vi "Actor Core.vi"(8 "error in":errorcluster, 11 "HIJ Multiple Cams App Demo In":refnum<class "HIJ Multiple Cams App Demo.lvclass">) -> (0 "error out":errorcluster, 3 "Actor out":refnum<class "Actor.lvclass">)   [LabVIEW 2014, in "HIJ Multiple Cams App Demo.lvlib" / "HIJ Multiple Cams App Demo.lvclass"]
doc: "(<B>Filename</B>: Actor Framework.lvlib:Actor.lvclass:Actor Core.vi)\n\nReceives messages to the actor, reacts to them, and initiates any error handling that may shut the actor down.\n\nDescendant classes may override this VI to append parallel tasks for the actor to complete while it handles messages. Overrides use the Call Parent Method node."
uses:
  HIJ Multiple Cams App Demo.lvclass
  <vilib>/ActorFramework/Actor/Actor.lvclass
  Applications/HIJ Single Cam App Demo/HIJ Single Cam App Demo/HIJ Single Cam App Demo.lvclass
  HIJ Multiple Cams App Demo Messages/Results from Cam 1 Msg/Results from Cam 1 Msg.lvclass
  HIJ Multiple Cams App Demo Messages/Results from Cam 2 Msg/Results from Cam 2 Msg.lvclass
  Shared Code/Viewable Actor/ViewableActor/ViewableActor.lvclass/ViewableActor.ctl
  HIJ Multiple Cams App Demo.lvclass/HIJ Multiple Cams App Demo.ctl
  Applications/HIJ Single Cam App Demo/HIJ Single Cam App Demo/HIJ Single Cam App Demo.lvclass/HIJ Single Cam App Demo.ctl
  Shared Code/Viewable Actor/ViewableActor Messages/Insert Into SubPanel Msg/Insert Into SubPanel Msg.lvclass/Insert Into SubPanel Msg.ctl
  <vilib>/ActorFramework/Message Enqueuer/Message Enqueuer.lvclass/Message Enqueuer.ctl
  <vilib>/ActorFramework/Actor/Actor.lvclass/Actor.ctl
  Applications/HIJ Vision Camera App/HIJ Vision Camera App Messages/Menu Selection Msg/Menu Selection Msg.lvclass/Menu Selection Msg.ctl
  Shared Code/Viewable Actor/ViewableActor/Write UI VI Ref.vi
  Applications/HIJ Single Cam App Demo/HIJ Single Cam App Demo/Write Caller Menu Ref.vi
  Applications/HIJ Single Cam App Demo/HIJ Single Cam App Demo/Write Publish Analyze Results Msg.vi
  <vilib>/ActorFramework/Message Enqueuer/Enqueue.vi
  <vilib>/ActorFramework/Message Enqueuer/Init from Existing Queue.vi
  Applications/HIJ Vision Camera App/HIJ Vision Camera App/Write my WorkDir.vi
  Applications/HIJ Vision Camera App/HIJ Vision Camera App/Write my ConfigDir.vi
  Applications/HIJ Vision Camera App/HIJ Vision Camera App/Write Start Camera.vi
  Applications/HIJ Vision Camera App/HIJ Vision Camera App/Write Start Acquisition.vi
  <vilib>/ActorFramework/Message Priority Queue/Priority Enqueue.vi
  Shared Code/Viewable Actor/ViewableActor Messages/Insert Into SubPanel Msg/Insert Into SubPanel Msg.lvclass
  <vilib>/ActorFramework/Message Enqueuer/Message Enqueuer.lvclass
  Applications/HIJ Vision Camera App/HIJ Vision Camera App Messages/Menu Selection Msg/Menu Selection Msg.lvclass
  <vilib>/ActorFramework/Stop Msg/Stop Msg.lvclass
  Shared Code/Viewable Actor/ViewableActor/ViewableActor.lvclass
panel:
  in  "Stop Button":bool
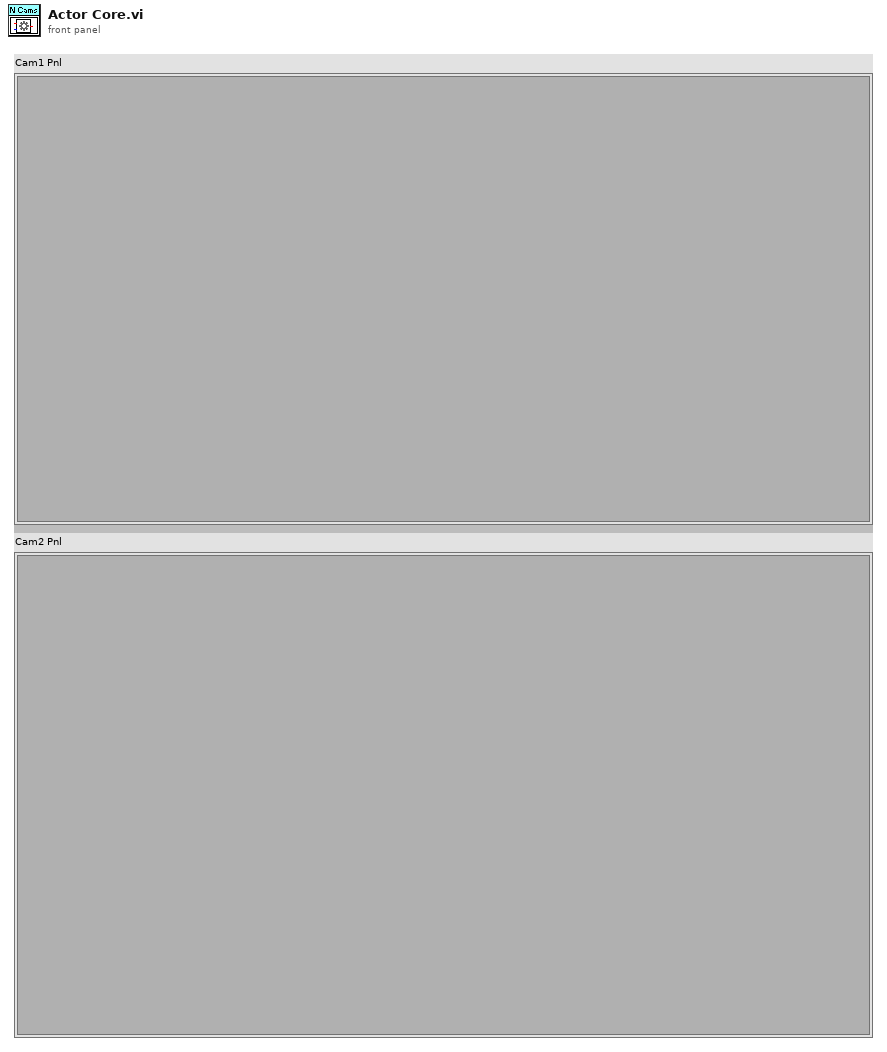
[diagram p1: front panel]
types:
  T1 = typedef "IMAQdx.ctl" = refnum<k21>
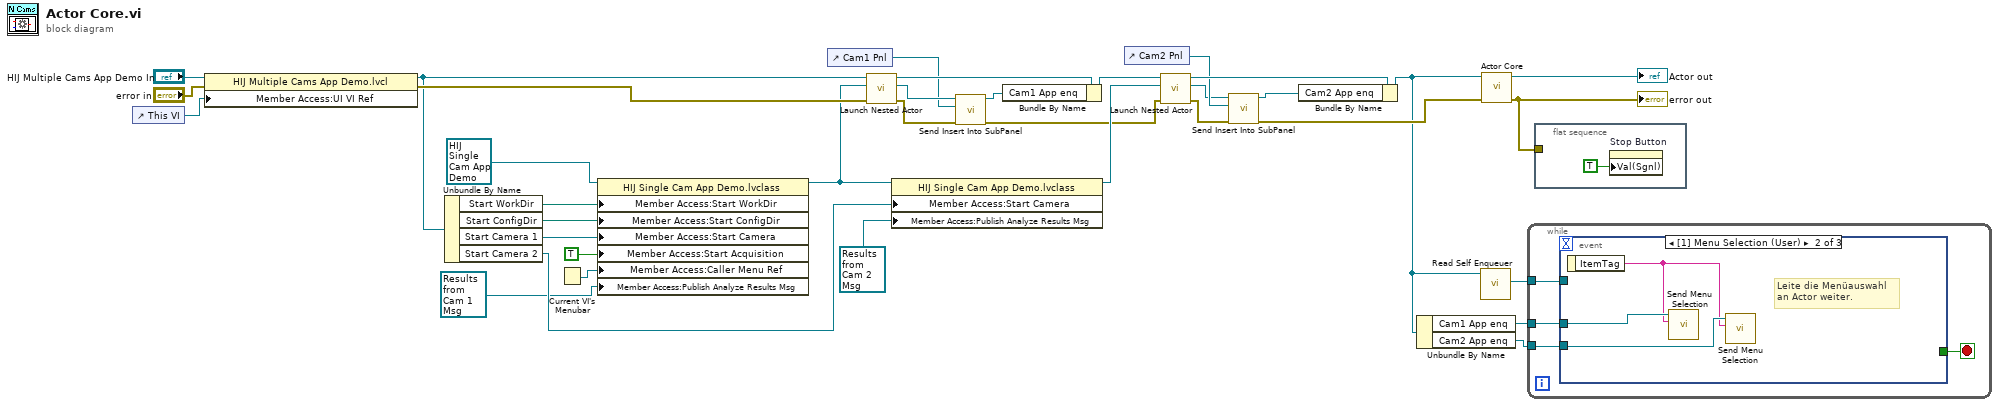
[diagram p0: block diagram]
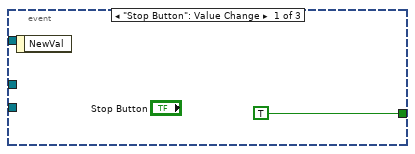
[diagram p2: hidden frame]
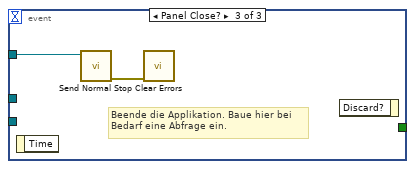
[diagram p3: hidden frame]
diagram:
  n1 = control-ref of="This VI"() -> (w30:refnum<vi>)
  n2 = property class="HIJ Multiple Cams App Demo.lvcl"(reference="HIJ Multiple Cams App Demo In", error in="error in", "Member Access:UI VI Ref"=w30) -> (reference out=w18:refnum<class "HIJ Multiple Cams App Demo.lvclass">, error out=w27:errorcluster)
  n3 = Unbundle By Name(w18) -> ("Start WorkDir"=w15:path, "Start ConfigDir"=w16:path, "Start Camera 1"=w17:T1, "Start Camera 2"=w14:T1)
  n4 = Current VI's Menubar() -> (w11:refnum<k9>)
  n5 = property class="HIJ Single Cam App Demo.lvclass"(reference=refnum<class "HIJ Single Cam App Demo.lvclass"> refnum ("HIJ Single Cam App Demo.lvlib:HIJ Single Cam App Demo.lvclass"), "Member Access:Start WorkDir"=w15, "Member Access:Start ConfigDir"=w16, "Member Access:Start Camera"=w17, "Member Access:Start Acquisition"=TRUE ("Start Acquisition"), "Member Access:Caller Menu Ref"=w11, "Member Access:Publish Analyze Results Msg"=refnum<class "Results from Cam 1 Msg.lvclass"> refnum ("HIJ Multiple Cams App Demo.lvlib:Results from Cam 1 Msg.lvclass")) -> (reference out=w26:refnum<class "HIJ Single Cam App Demo.lvclass">)  [unwired: 1 in, 1 out]
  n6 = control-ref of="Cam1 Pnl"() -> (w19:refnum<vi>)
  n7 = call <vilib>:"Launch Nested Actor.vi"("error in (no error)"=w27, "Nested Actor"=w26, "Caller Actor in"=w18) -> ("error out"=w22:errorcluster, "Nested Actor's Enqueuer"=w24:refnum<class "Message Enqueuer.lvclass">, "Caller Actor out"=w23:refnum<class "HIJ Multiple Cams App Demo.lvclass">)  [unwired: 6 in]
  n8 = property class="HIJ Single Cam App Demo.lvclass"(reference=w26, "Member Access:Start Camera"=w14, "Member Access:Publish Analyze Results Msg"=refnum<class "Results from Cam 2 Msg.lvclass"> refnum ("HIJ Multiple Cams App Demo.lvlib:Results from Cam 2 Msg.lvclass")) -> (reference out=w25:refnum<class "HIJ Single Cam App Demo.lvclass">)  [unwired: 1 in, 1 out]
  n9 = call "Send Insert Into SubPanel.vi"("error in (no error)"=w22, "SubPanel Ref"=w19, "Message Enqueuer"=w24) -> ("error out"=w21:errorcluster, "Message Enqueuer out"=w12:refnum<class "Message Enqueuer.lvclass">)  [unwired: 7 in]
  n10 = Bundle By Name(cluster=w23, "Cam1 App enq"=w12) -> (w13:refnum<class "HIJ Multiple Cams App Demo.lvclass">)
  n11 = control-ref of="Cam2 Pnl"() -> (w8:refnum<vi>)
  n12 = call <vilib>:"Launch Nested Actor.vi"("error in (no error)"=w21, "Nested Actor"=w25, "Caller Actor in"=w13) -> ("error out"=w9:errorcluster, "Nested Actor's Enqueuer"=w7:refnum<class "Message Enqueuer.lvclass">, "Caller Actor out"=w10:refnum<class "HIJ Multiple Cams App Demo.lvclass">)  [unwired: 6 in]
  n13 = call "Send Insert Into SubPanel.vi"("error in (no error)"=w9, "SubPanel Ref"=w8, "Message Enqueuer"=w7) -> ("error out"=w20:errorcluster, "Message Enqueuer out"=w6:refnum<class "Message Enqueuer.lvclass">)  [unwired: 7 in]
  n14 = Bundle By Name(cluster=w10, "Cam2 App enq"=w6) -> (w5:refnum<class "HIJ Multiple Cams App Demo.lvclass">)
  n15 = Unbundle By Name(w5) -> ("Cam1 App enq"=w4:refnum<class "Message Enqueuer.lvclass">, "Cam2 App enq"=w3:refnum<class "Message Enqueuer.lvclass">)
  n16 = call <vilib>:"Read Self Enqueuer.vi"("Actor"=w5) -> ("Self Enqueuer"=w33:refnum<class "Message Enqueuer.lvclass">)  [unwired: 10 in]
  n17 = call-parent "Actor Core.vi"("error in"=w20, "Actor in"=w5) -> ("error out"=w34:errorcluster, "Actor out"=→"Actor out":refnum<class "Actor.lvclass">)  [unwired: 8 in]
  "error out" <- w34
  n18 = while {
    tunnel: w33 -> [w38]
    tunnel: w4 -> [w37]
    tunnel: w3 -> [w36]
    stop <- w39 stop-if-true
    n19 = event shown="[1] Menu Selection (User)" {
      selector: _ -> [_ _ _]
      dyn-events: _ -> [_ _ _]
      timeout: _ -> [_ _ _]
      tunnel: [TRUE _ _] -> w39
      tunnel: w38 -> [_ _ w45]
      tunnel: w37 -> [_ w43 _]
      tunnel: w36 -> [_ w42 _]
      event "Stop Button": Value Change {
        n20 = event-data() -> ()  [unwired: 1 in, 1 out]
      }
      event Menu Selection (User) {
        # "Leite die Menüauswahl \nan Actor weiter."
        n21 = event-data() -> ("ItemTag"=w41:string)  [unwired: 1 in]
        n22 = call "Send Menu Selection.vi"("MenuTag"=w41, "Message Enqueuer"=w43) -> ()  [unwired: 8 in, 2 out]
        n23 = call "Send Menu Selection.vi"("MenuTag"=w41, "Message Enqueuer"=w42) -> ()  [unwired: 8 in, 2 out]
      }
      event Panel Close? {
        # "Beende die Applikation. Baue hier bei\nBedarf eine Abfrage ein."
        n24 = event-data() -> ()  [unwired: 1 in, 1 out]
        n25 = call <vilib>:"Send Normal Stop.vi"("Message Enqueuer"=w45) -> ("error out"=w44:errorcluster)  [unwired: 10 in]
        n26 = call <vilib>:"Clear Errors.vi"("error in (no error)"=w44) -> ()  [unwired: 5 in, 2 out]
        n27 = event-data() -> ()  [unwired: 2 in, 1 out]
      }
    }
  }
  n28 = flat-sequence {
    tunnel: w34 -> [_]
    frame #0 {
      n29 = property on="Stop Button" class="Bool (strict)"("Val(Sgnl)"=TRUE) -> ()  [unwired: 2 in, 2 out]
    }
  }
